vi "Find Blobs.vi"(11 "Image In":T1) -> (2 "Blob Data":T2, 3 "Image Out":T1)   [LabVIEW 2015]
uses:
  <vilib>/vision/Image Controls.llb/IMAQ Image.ctl
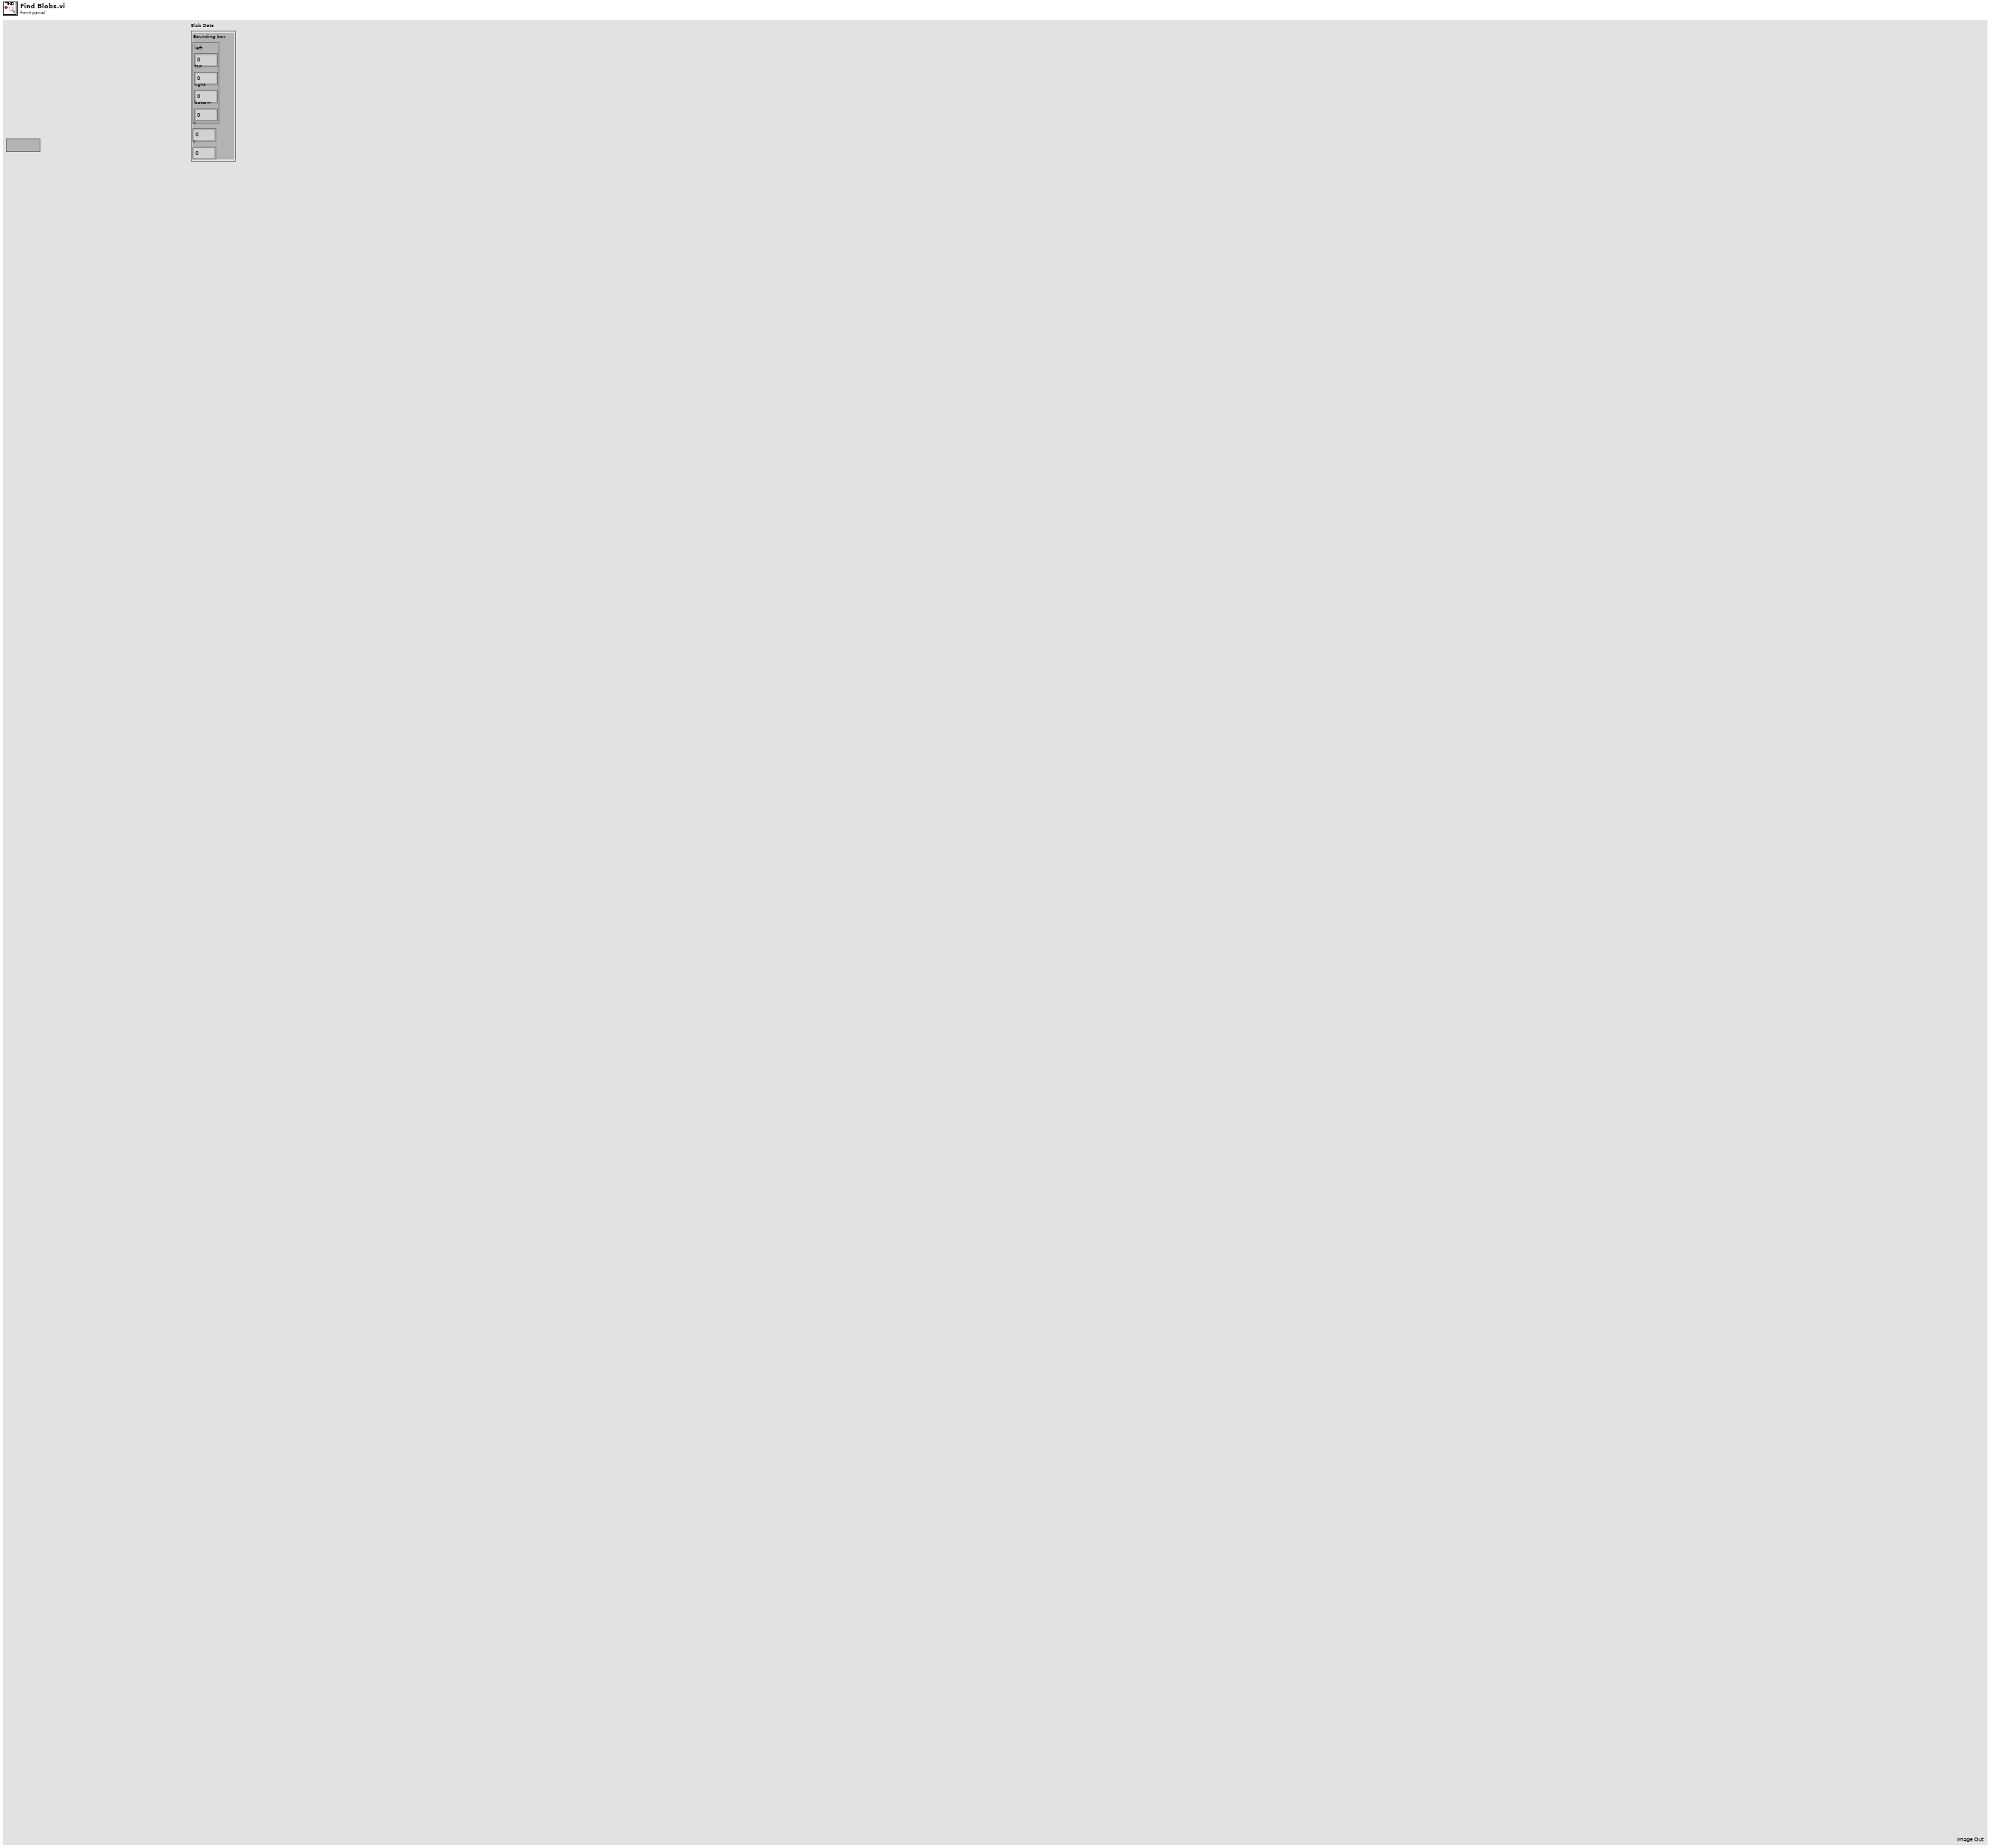
[diagram p1: front panel]
types:
  T1 = typedef "IMAQ Image.ctl" = refnum<image>
  T2 = cluster{"Bounding box":cluster{"left":dbl, "top":dbl, "right":dbl, "bottom":dbl}, "x":dbl, "y":dbl}
  T3 = typedef "Particle Parameters" = i32
  T4 = cluster{"Bounding box":cluster{"left":dbl, "top":dbl, "right":dbl, "bottom":dbl}, "Aspect Ratio":dbl, "Area to CH":dbl, "X Mask":dbl, "Y Mask":dbl, "Moment":dbl, "x":dbl, "y":dbl}[]
  T5 = cluster{"Bounding box":cluster{"left":dbl, "top":dbl, "right":dbl, "bottom":dbl}, "Aspect Ratio":dbl, "Area to CH":dbl, "X Mask":dbl, "Y Mask":dbl, "Moment":dbl, "x":dbl, "y":dbl}
  T6 = cluster{"left":dbl, "top":dbl, "right":dbl, "bottom":dbl}
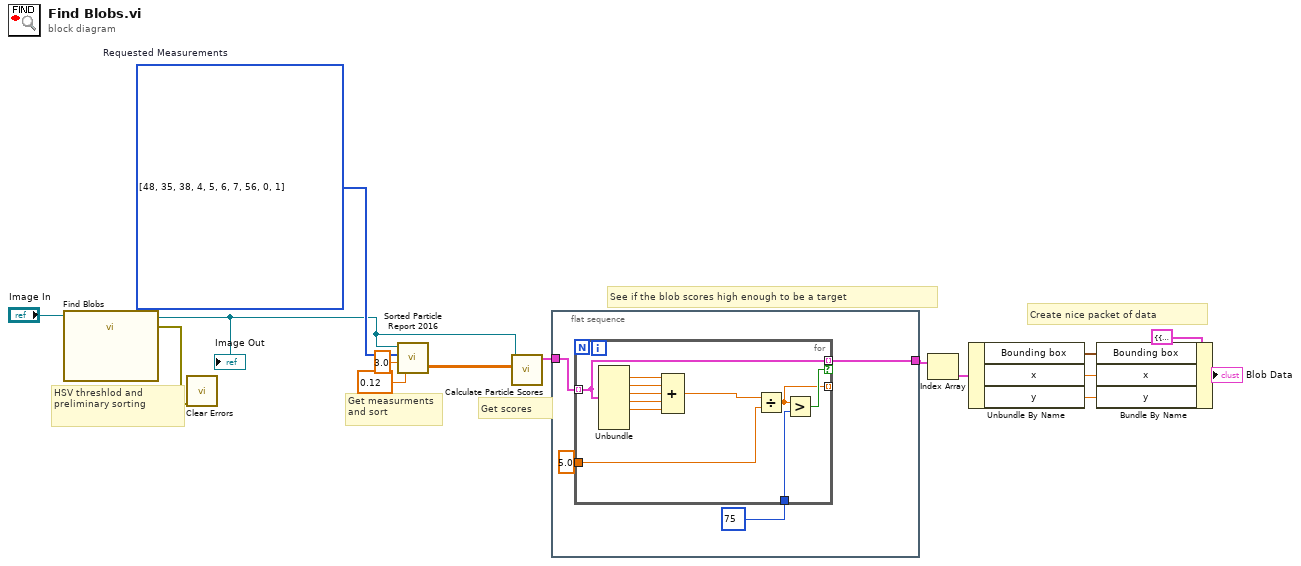
[diagram p0: block diagram]
diagram:
  w15 = T3[] [48, 35, 38, 4, 5, 6, 7, 56, 0, 1] items=["Center of Mass X", "Center of Mass Y", "First Pixel X", "First Pixel Y", "Bounding Rect Left", "Bounding Rect Top", "Bounding Rect Right", "Bounding Rect Bottom", "Max Feret Diameter Start X", "Max Feret Diameter Start Y", "Max Feret Diameter End X", "Max Feret Diameter End Y", "Max Horiz. Segment Length Left", "Max Horiz. Segment Length Right", "Max Horiz. Segment Length Row", "-", "Bounding Rect Width", "Bounding Rect Height", "Bounding Rect Diagonal", "Perimeter", "Convex Hull Perimeter", "Holes' Perimeter", "Max Feret Diameter", "Equivalent Ellipse Major Axis", "Equivalent Ellipse Minor Axis", "Equivalent Ellipse Minor Axis (Feret)", "Equivalent Rect Long Side", "Equivalent Rect Short Side", "Equivalent Rect Diagonal", "Equivalent Rect Short Side (Feret)", "Average Horiz. Segment Length", "Average Vert. Segment Length", "Hydraulic Radius", "Waddel Disk Diameter", "-", "Area", "Holes' Area", "Particle & Holes' Area", "Convex Hull Area", "Image Area", "-", "Number of Holes", "Number of Horiz. Segments", "Number of Vert. Segments", "-", "Orientation", "Max Feret Diameter Orientation", "-", "% Area/Image Area", "% Area/(Particle & Holes' Area)", "Ratio of Equivalent Ellipse Axes", "Ratio of Equivalent Rect Sides", "-", "Elongation Factor", "Compactness Factor", "Heywood Circularity Factor", "Type Factor", "-", "Sum X", "Sum Y", "Sum XX", "Sum XY", "Sum YY", "Sum XXX", "Sum XXY", "Sum XYY", "Sum YYY", "-", "Moment of Inertia XX", "Moment of Inertia XY", "Moment of Inertia YY", "Moment of Inertia XXX", "Moment of Inertia XXY", "Moment of Inertia XYY", "Moment of Inertia YYY", "Norm. Moment of Inertia XX", "Norm. Moment of Inertia XY", "Norm. Moment of Inertia YY", "Norm. Moment of Inertia XXX", "Norm. Moment of Inertia XXY", "Norm. Moment of Inertia XYY", "Norm. Moment of Inertia YYY", "Hu Moment 1", "Hu Moment 2", "Hu Moment 3", "Hu Moment 4", "Hu Moment 5", "Hu Moment 6", "Hu Moment 7"]  # Requested Measurements
  # "Create nice packet of data"
  # "See if the blob scores high enough to be a target"
  # "Get scores"
  # "Get measurments\nand sort"
  # "HSV threshlod and \npreliminary sorting"
  n1 = call "Find Blobs"("Image In"="Image In") -> ("Image Out"=w11:T1, "error out"=w1:errorcluster)  [unwired: 23 in, 2 out]
  "Image Out" <- w11
  n2 = call <vilib>:"Clear Errors.vi"("error in (no error)"=w1) -> ()  [unwired: 5 in, 2 out]
  n3 = call "Sorted Particle Report 2016.vi"("Min Area Size %"=0.12, "Particle Count Limit"=3.0, "Pixel Measurements"=w15, "Image in"=w11) -> ("Sorted Data"=w12:dbl[][])  [unwired: 1 out]
  n4 = call "Calculate Particle Scores.vi"("Sorted Data"=w12, "Image in"=w11) -> ("Scores"=w10:T4)  [unwired: 9 in]
  n5 = flat-sequence {
    tunnel: w10 -> [w19]
    tunnel: [w18] -> w8
    frame #0 {
      n6 = for {
        tunnel: w19 -> [w28] mode=indexing
        tunnel: [w28] -> w18 mode=indexing if=w27
        tunnel: [w26] -> _ mode=indexing
        tunnel: 75 ("Min Score Threshold") -> [w20]
        tunnel: 5.0 ("y") -> [w21]
        n7 = Unbundle(w28) -> ("Aspect Ratio"=w30:dbl, "Area to CH"=w29:dbl, "X Mask"=w23:dbl, "Y Mask"=w24:dbl, "Moment"=w25:dbl)  [unwired: 3 out]
        n8 = Compound Arithmetic op=ADD(w30, w29, w23, w24, w25) -> (w22:dbl)
        n9 = Divide(x=w22, y=w21) -> (x/y=w26:dbl)
        n10 = Greater?(x=w26, y=w20) -> (0:w27:bool)
      }
    }
  }
  n11 = Index Array(array=w8) -> (element=w7:T5)  [unwired: 1 in]
  n12 = Unbundle By Name(w7) -> ("Bounding box"=w6:T6, "x"=w5:dbl, "y"=w4:dbl)
  n13 = Bundle By Name(cluster=T2 {"Bounding box"={"left"=0.0, "top"=0.0, "right"=0.0, "bottom"=0.0}, "x"=0.0, "y"=0.0} ("input cluster"), "Bounding box"=w6, "x"=w5, "y"=w4) -> (→"Blob Data":T2)
